vi "Evaluate Key Down Event.vi"(9 "PlatMods":T2, 10 "Char":i16, 11 "VKey":T1) -> (3 "do forward":bool)   [LabVIEW 2020, in "UI Manager.lvlib"]
doc: "Evaluates the key down events and decides which ones to forward.\n\nCurrently we only process those key presses that are necessary for invoking our \"Help Provider\" (see https://dokuwiki.hampel-soft.com/code/hse-labs/help-provider). In the future, these should be configurable.\n\n____\nHAMPEL SOFTWARE ENGINEERING v2.6.0 (2023-12-19 10:54)"
uses:
  UI Manager.lvlib
  <vilib>/event_ctls.llb/eventvkey.ctl
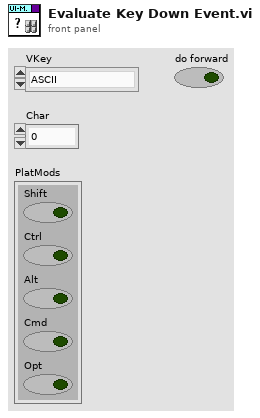
[diagram p1: front panel]
types:
  T1 = typedef "eventvkey.ctl" = enum16{"ASCII", "Enter", "Return", "Shift", "Ctrl", "Alt", "Cmd", "Opt", "Caps", "NumLock", "Clear", "Break", "Up", "Down", "Left", "Right", "Insert", "Delete", "Home", "End", "PageUp", "PageDown", "Escape", "Help", "Pause", "ScrollLock", "F1", "F2", "F3", "F4", "F5", "F6", "F7", "F8", "F9", "F10", "F11", "F12", "F13", "F14", "F15", "F16", "F17", "F18", "F19", "F20", "F21", "F22", "F23", "F24", "Play", "VolumeUp", "VolumeDown", "Mute", "Two Byte Char"}
  T2 = cluster{"Shift":bool, "Ctrl":bool, "Alt":bool, "Cmd":bool, "Opt":bool}
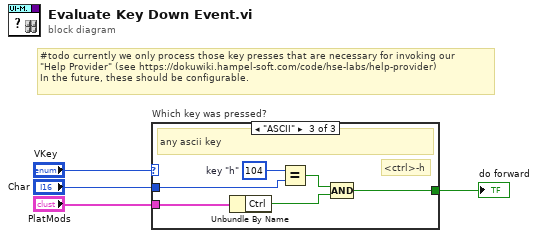
[diagram p0: block diagram]
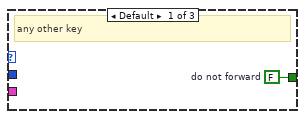
[diagram p2: hidden frame]
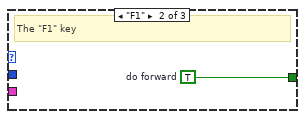
[diagram p3: hidden frame]
diagram:
  # "#todo currently we only process those key presses that are necessary for invoking our \n\"Help Provider\" (see https://dokuwiki.hampel-soft.com/code/hse-labs/help-provider)\nIn the future, these should be configurable."
  n1 = case "Which key was pressed?" shown="\"ASCII\"" "VKey" {
    tunnel: "PlatMods" -> [_ _ w10]
    tunnel: "Char" -> [_ _ w11]
    tunnel: [w5 w6 w7] -> w1
    frame Default {
      w5 = FALSE  # do not forward
      # "any other key"
    }
    frame "F1" {
      w6 = TRUE  # do forward
      # "The \"F1\" key"
    }
    frame "ASCII" {
      w12 = i16 104  # key "h"
      # "<ctrl>-h"
      # "any ascii key"
      n2 = Unbundle By Name(w10) -> ("Ctrl"=w8:bool)
      n3 = Equal?(x=w12, y=w11) -> (x = y?=w9:bool)
      n4 = Compound Arithmetic op=AND(w9, w8) -> (w7:bool)
    }
  }
  "do forward" <- w1
